vi "Prepare for a Scan_Load Settings.vi"(8 "error in (no error)":errorcluster, 11 "Command IN":string) -> (0 "error out":errorcluster)   [LabVIEW 2012]
doc: "SciScan 1.2 160622"
uses:
  INI/settingsIO/Settings IO_Commands.ctl
  MacroGUI Module/SubVIs/FGV_Macro Settings to GFG_Command.ctl
  Custom Controls/scan mode main settings tab.ctl
  image & display/Draw ROI on Line Scan Display Command.ctl
  Custom Controls/MAIN Image panel tab Control type def.ctl
  Custom Controls/advanced settings inner tab CTL.ctl
  System.Windows.Forms
panel:
  in  "Updating Settings...":refnum<k24>(container)
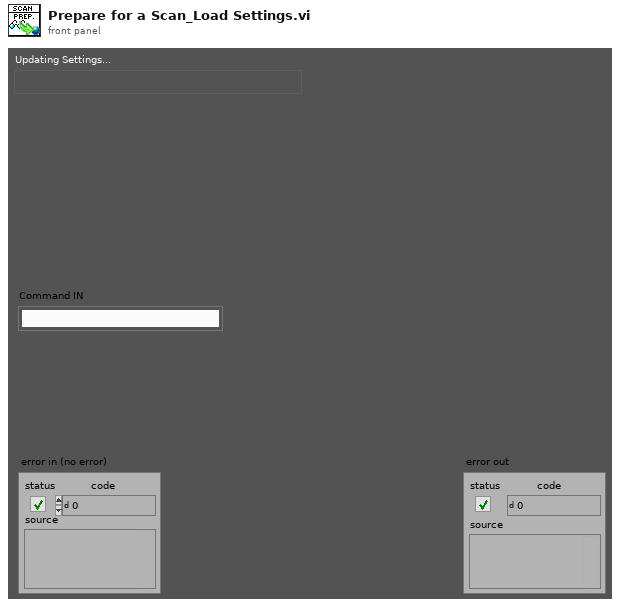
[diagram p1: front panel]
types:
  T1 = typedef "Setting File Types.ctl" = enum16{"2D.Frame.Scan.Settings", "2D.Line.Scan.Settings", "Z.Stack.Settings", "HW Settings", "Configuration Settings", "Unknown Settings", "Fast.Z.Settings"}
  T2 = typedef "scan mode main settings tab.ctl" = enum32{"2D frame", "2D line scan", "general settings", "Z Stack", "piezo"}
  T3 = typedef "FGV_Macro Settings to GFG_Command.ctl" = enum16{"Get Current Settings", "Backup Curent Settings", "Recover Backed up settings", "Overwrite Current Settings"}
  T4 = typedef "Settings IO_Commands.ctl" = enum16{"Write HW Settings", "Write Config Settings", "Read HW Settings", "Read Config Settings", "Write Line-Scan Settings", "Write Frame-Scan Settings", "Write Z-Stack Settings", "Read Line-Scan Settings", "Read Frame-Scan Settings", "Read Z-Stack Settings", "Read Fast-Z Settings", "Write Fast-Z Settings"}
  T5 = typedef "MAIN Image panel tab Control type def.ctl" = enum32{"Channel 1", "Channel 2", "Channel 3", "Channel 4", "all channels", "RGB overlay", "ROI", "arbitrary line scan"}
  T6 = typedef "Draw ROI on Line Scan Display Command.ctl" = enum16{"Draw ROI from GFG", "Clear ROI"}
  T7 = enum16{"Always Generate", "Generate if no valid image"}
  T8 = typedef "advanced settings inner tab CTL.ctl" = enum32{"arb. frames", "AO", "AI", "channels", "trigger", "Zstack data"}
  T9 = typedef "GFG Variable for IO.ctl" = cluster{"Variable Name":string, "Value (Variant)":variant, "data type":string}
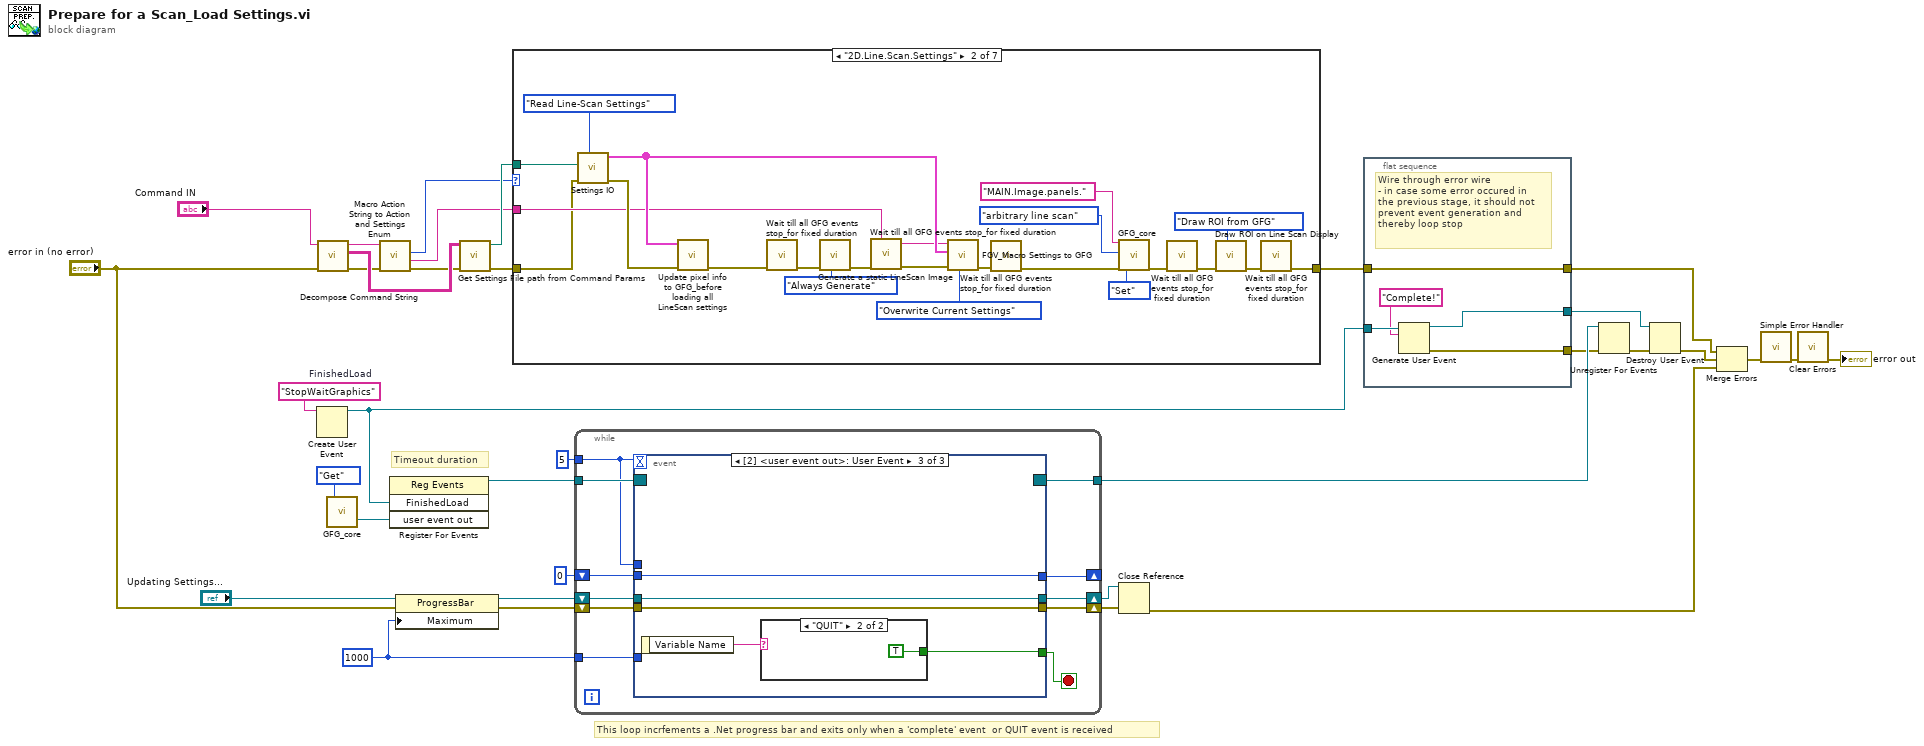
[diagram p0: block diagram]
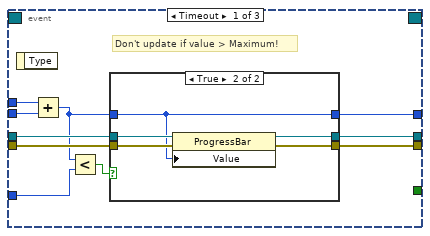
[diagram p2: hidden frame]
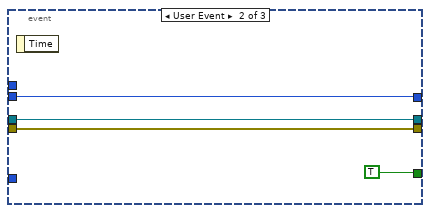
[diagram p4: hidden frame]
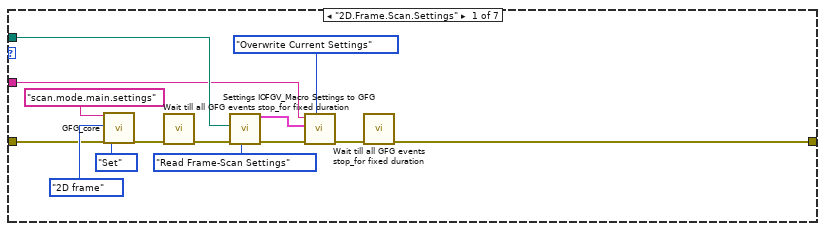
[diagram p6: hidden frame]
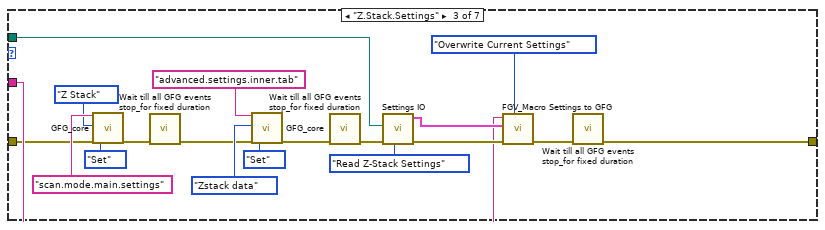
[diagram p7: hidden frame]
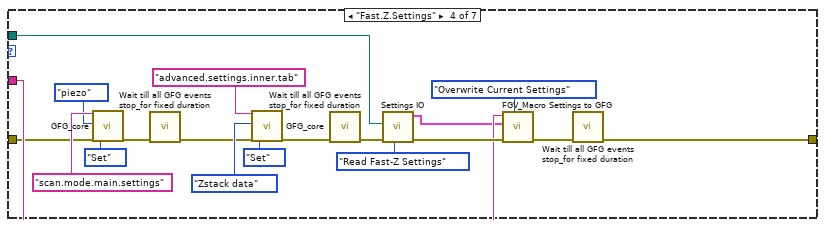
[diagram p8: hidden frame]
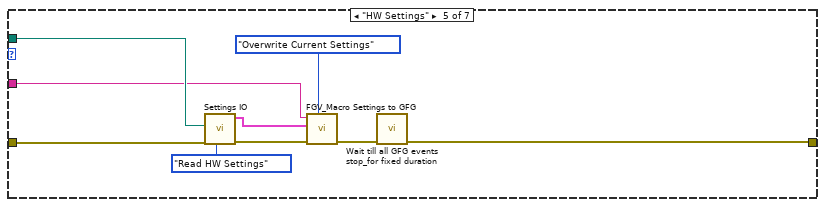
[diagram p9: hidden frame]
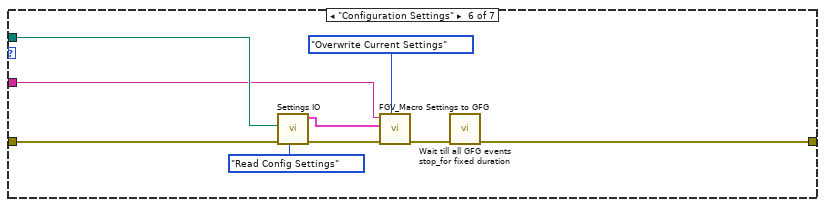
[diagram p10: hidden frame]
diagram:
  w12 = 1000 ("Maximum")
  w25 = "StopWaitGraphics"  # FinishedLoad
  # "This loop incrfements a .Net progress bar and exits only when a 'complete' event  or QUIT event is received"
  # "Timeout duration"
  n1 = Create User Event(user event datatype=w25) -> (user event=w22:refnum<user-event>)  [unwired: 1 in, 1 out]
  n2 = call "Decompose Command String.vi"("Error In"="error in (no error)", "Command IN"="Command IN") -> ("Error Out"=w33:errorcluster, "Parameter Table"=w34:string[][], "Action"=w32:string)  [unwired: 6 in, 1 out]
  n3 = call "GFG_core.vi"("Action"=enum16{"Init", "Set", "Get", "Clear"}."Get") -> ("user event out"=w1:refnum<user-event>)  [unwired: 12 in, 6 out]
  n4 = call "Macro Action String to Action and Settings Enum.vi"("error in (no error)"=w33, "Action String IN"=w32) -> ("error out"=w31:errorcluster, "Settings File Type OUT (String)"=w29:string, "Setting File Type OUT"=w28:T1)  [unwired: 6 in, 1 out]
  n5 = register-events(w22, w1) -> (reference out=w21:refnum<event-registration>)  [unwired: 2 in, 1 out]
  n6 = property class="ProgressBar"(reference="Updating Settings...", error in="error in (no error)", "Maximum"=w12) -> (reference out=w19:refnum<k24>, error out=w20:errorcluster)
  n7 = call "Get Settings File path from Command Params.vi"("error in (no error)"=w31, "Params Array IN"=w34) -> ("error out"=w26:errorcluster, "Settings Path OUT"=w30:path)  [unwired: 8 in]
  n8 = case shown="\"2D.Line.Scan.Settings\"" w28 {
    tunnel: [w43 w49 w82 w91 w109 w120 w127] -> w9
    tunnel: w30 -> [w42 w53 w84 w104 w111 w119 _]
    tunnel: w29 -> [w41 w52 w85 w105 w110 w118 _]
    tunnel: w26 -> [w37 w51 w75 w96 w112 w121 w127]
    frame "2D.Frame.Scan.Settings" {
      n9 = call "GFG_core.vi"("Variable Name in"="scan.mode.main.settings", "Variant in"=scan_mode_main_settings_tab."2D frame" ("scan mode main settings"), "error in (no error)"=w37, "Action"=enum16{"Init", "Set", "Get"}."Set") -> ("error out"=w36:errorcluster)  [unwired: 9 in, 6 out]
      n10 = call "Wait till all GFG events stop_for fixed duration.vi"("error in (no error)"=w36) -> ("error out"=w35:errorcluster)  [unwired: 10 in]
      n11 = call "Settings IO.vi"("SettingsFileIO_Commands"=Settings_IO_Commands."Read Frame-Scan Settings", "Error In"=w35, "File Path (for scan specific settings)"=w42) -> ("Error Out"=w46:errorcluster, "Settings Array OUT"=w45:T9[])  [unwired: 6 in, 1 out]
      n12 = call "FGV_Macro Settings to GFG.vi"("FGV_Macro Settings to GFG_Command"=FGV_Macro_Settings_to_GFG_Command."Overwrite Current Settings", "error in (no error)"=w46, "New Settings IN"=w45, "Settings type string IN"=w41) -> ("error out"=w44:errorcluster)  [unwired: 5 in, 2 out]
      n13 = call "Wait till all GFG events stop_for fixed duration.vi"("error in (no error)"=w44) -> ("error out"=w43:errorcluster)  [unwired: 10 in]
    }
    frame "2D.Line.Scan.Settings" {
      n14 = call "Settings IO.vi"("SettingsFileIO_Commands"=Settings_IO_Commands."Read Line-Scan Settings", "Error In"=w51, "File Path (for scan specific settings)"=w53) -> ("Error Out"=w68:errorcluster, "Settings Array OUT"=w67:T9[])  [unwired: 6 in, 1 out]
      n15 = call "Update pixel info to GFG_before loading all LineScan settings.vi"("error in (no error)"=w68, "All LineScan Settings IN"=w67) -> ("error out"=w66:errorcluster)  [unwired: 9 in]
      n16 = call "Wait till all GFG events stop_for fixed duration.vi"("error in (no error)"=w66) -> ("error out"=w64:errorcluster)  [unwired: 10 in]
      n17 = call "Generate a static LineScan Image.vi"("Generate Static Image Options"=T7."Always Generate", "error in (no error)"=w64) -> ("error out"=w59:errorcluster)  [unwired: 9 in]
      n18 = call "Wait till all GFG events stop_for fixed duration.vi"("error in (no error)"=w59) -> ("error out"=w58:errorcluster)  [unwired: 10 in]
      n19 = call "FGV_Macro Settings to GFG.vi"("FGV_Macro Settings to GFG_Command"=FGV_Macro_Settings_to_GFG_Command."Overwrite Current Settings", "error in (no error)"=w58, "New Settings IN"=w67, "Settings type string IN"=w52) -> ("error out"=w57:errorcluster)  [unwired: 5 in, 2 out]
      n20 = call "Wait till all GFG events stop_for fixed duration.vi"("error in (no error)"=w57) -> ("error out"=w54:errorcluster)  [unwired: 10 in]
      n21 = call "GFG_core.vi"("Variable Name in"="MAIN.Image.panels.", "Variant in"=MAIN_Image_panel_tab_Control_type_def."arbitrary line scan" ("MAIN Image panels"), "error in (no error)"=w54, "Action"=enum16{"Init", "Set", "Get"}."Set") -> ("error out"=w56:errorcluster)  [unwired: 9 in, 6 out]
      n22 = call "Wait till all GFG events stop_for fixed duration.vi"("error in (no error)"=w56) -> ("error out"=w55:errorcluster)  [unwired: 10 in]
      n23 = call "Draw ROI on Line Scan Display.vi"("Draw ROI on Line Scan Display_Command"=Draw_ROI_on_Line_Scan_Display_Command."Draw ROI from GFG", "error in (no error)"=w55) -> ("error out"=w50:errorcluster)  [unwired: 9 in]
      n24 = call "Wait till all GFG events stop_for fixed duration.vi"("error in (no error)"=w50) -> ("error out"=w49:errorcluster)  [unwired: 10 in]
    }
    frame "Z.Stack.Settings" {
      n25 = call "GFG_core.vi"("Variable Name in"="scan.mode.main.settings", "Variant in"=scan_mode_main_settings_tab."Z Stack" ("scan mode main settings"), "error in (no error)"=w75, "Action"=enum16{"Init", "Set", "Get"}."Set") -> ("error out"=w72:errorcluster)  [unwired: 9 in, 6 out]
      n26 = call "Wait till all GFG events stop_for fixed duration.vi"("error in (no error)"=w72) -> ("error out"=w73:errorcluster)  [unwired: 10 in]
      n27 = call "GFG_core.vi"("Variable Name in"="advanced.settings.inner.tab", "Variant in"=advanced_settings_inner_tab_CTL."Zstack data" ("advanced settings inner tab"), "error in (no error)"=w73, "Action"=enum16{"Init", "Set", "Get"}."Set") -> ("error out"=w74:errorcluster)  [unwired: 9 in, 6 out]
      n28 = call "Wait till all GFG events stop_for fixed duration.vi"("error in (no error)"=w74) -> ("error out"=w71:errorcluster)  [unwired: 10 in]
      n29 = call "Settings IO.vi"("SettingsFileIO_Commands"=Settings_IO_Commands."Read Z-Stack Settings", "Error In"=w71, "File Path (for scan specific settings)"=w84) -> ("Error Out"=w87:errorcluster, "Settings Array OUT"=w86:T9[])  [unwired: 6 in, 1 out]
      n30 = call "FGV_Macro Settings to GFG.vi"("FGV_Macro Settings to GFG_Command"=FGV_Macro_Settings_to_GFG_Command."Overwrite Current Settings", "error in (no error)"=w87, "New Settings IN"=w86, "Settings type string IN"=w85) -> ("error out"=w83:errorcluster)  [unwired: 5 in, 2 out]
      n31 = call "Wait till all GFG events stop_for fixed duration.vi"("error in (no error)"=w83) -> ("error out"=w82:errorcluster)  [unwired: 10 in]
    }
    frame "Fast.Z.Settings" {
      n32 = call "GFG_core.vi"("Variable Name in"="scan.mode.main.settings", "Variant in"=scan_mode_main_settings_tab."piezo" ("scan mode main settings"), "error in (no error)"=w96, "Action"=enum16{"Init", "Set", "Get"}."Set") -> ("error out"=w93:errorcluster)  [unwired: 9 in, 6 out]
      n33 = call "Wait till all GFG events stop_for fixed duration.vi"("error in (no error)"=w93) -> ("error out"=w94:errorcluster)  [unwired: 10 in]
      n34 = call "GFG_core.vi"("Variable Name in"="advanced.settings.inner.tab", "Variant in"=advanced_settings_inner_tab_CTL."Zstack data" ("advanced settings inner tab"), "error in (no error)"=w94, "Action"=enum16{"Init", "Set", "Get"}."Set") -> ("error out"=w95:errorcluster)  [unwired: 9 in, 6 out]
      n35 = call "Wait till all GFG events stop_for fixed duration.vi"("error in (no error)"=w95) -> ("error out"=w92:errorcluster)  [unwired: 10 in]
      n36 = call "Settings IO.vi"("SettingsFileIO_Commands"=Settings_IO_Commands."Read Fast-Z Settings", "Error In"=w92, "File Path (for scan specific settings)"=w104) -> ("Error Out"=w106:errorcluster, "Settings Array OUT"=w90:T9[])  [unwired: 6 in, 1 out]
      n37 = call "FGV_Macro Settings to GFG.vi"("FGV_Macro Settings to GFG_Command"=FGV_Macro_Settings_to_GFG_Command."Overwrite Current Settings", "error in (no error)"=w106, "New Settings IN"=w90, "Settings type string IN"=w105) -> ("error out"=w103:errorcluster)  [unwired: 5 in, 2 out]
      n38 = call "Wait till all GFG events stop_for fixed duration.vi"("error in (no error)"=w103) -> ("error out"=w91:errorcluster)  [unwired: 10 in]
    }
    frame "HW Settings" {
      n39 = call "Settings IO.vi"("SettingsFileIO_Commands"=Settings_IO_Commands."Read HW Settings", "Error In"=w112, "File Path (for scan specific settings)"=w111) -> ("Error Out"=w115:errorcluster, "Settings Array OUT"=w114:T9[])  [unwired: 6 in, 1 out]
      n40 = call "FGV_Macro Settings to GFG.vi"("FGV_Macro Settings to GFG_Command"=FGV_Macro_Settings_to_GFG_Command."Overwrite Current Settings", "error in (no error)"=w115, "New Settings IN"=w114, "Settings type string IN"=w110) -> ("error out"=w113:errorcluster)  [unwired: 5 in, 2 out]
      n41 = call "Wait till all GFG events stop_for fixed duration.vi"("error in (no error)"=w113) -> ("error out"=w109:errorcluster)  [unwired: 10 in]
    }
    frame "Configuration Settings" {
      n42 = call "Settings IO.vi"("SettingsFileIO_Commands"=Settings_IO_Commands."Read Config Settings", "Error In"=w121, "File Path (for scan specific settings)"=w119) -> ("Error Out"=w124:errorcluster, "Settings Array OUT"=w123:T9[])  [unwired: 6 in, 1 out]
      n43 = call "FGV_Macro Settings to GFG.vi"("FGV_Macro Settings to GFG_Command"=FGV_Macro_Settings_to_GFG_Command."Overwrite Current Settings", "error in (no error)"=w124, "New Settings IN"=w123, "Settings type string IN"=w118) -> ("error out"=w122:errorcluster)  [unwired: 5 in, 2 out]
      n44 = call "Wait till all GFG events stop_for fixed duration.vi"("error in (no error)"=w122) -> ("error out"=w120:errorcluster)  [unwired: 10 in]
    }
    frame "Unknown Settings", Default {
    }
  }
  n45 = while {
    shift-right: [w137] -> _
    shift-left: 0 -> [w138]
    tunnel: 5 -> [w129]
    tunnel: w21 -> [w136]
    shift-right: [w132] -> w17
    shift-left: w20 -> [w133]
    shift-right: [w131] -> w16
    shift-left: w19 -> [w135]
    tunnel: w12 -> [w130]
    tunnel: [w128] -> w6
    stop <- w134 stop-if-true
    n46 = event shown="[2] <user event out>: User Event" {
      selector: w136 -> [_ _ _]
      dyn-events: [_ _ _] -> w128
      timeout: w129 -> [_ _ _]
      tunnel: w138 -> [w141 w159 w165]
      tunnel: [w142 w159 w165] -> w137
      tunnel: w135 -> [w148 w157 w163]
      tunnel: [_ TRUE w161] -> w134
      tunnel: w133 -> [w147 w158 w164]
      tunnel: [w146 w158 w164] -> w132
      tunnel: [w145 w157 w163] -> w131
      tunnel: w130 -> [w143 _ _]
      tunnel: w129 -> [w139 _ _]
      event Timeout {
        # "Don't update if value > Maximum!"
        n47 = event-data() -> ()  [unwired: 1 in, 1 out]
        n48 = Add(x=w139, y=w141) -> (x+y=w140:i32)
        n49 = Less?(x=w140, y=w143) -> (x < y?=w144:bool)
        n50 = case shown="True" w144 {
          tunnel: w148 -> [w150 w156]
          tunnel: w147 -> [w151 w155]
          tunnel: w140 -> [w149 w152]
          tunnel: [w151 w154] -> w146
          tunnel: [w150 w153] -> w145
          tunnel: [w149 w152] -> w142
          frame False {
          }
          frame True {
            n51 = property class="ProgressBar"(reference=w156, error in=w155, "Value"=w152) -> (reference out=w153:refnum<k24>, error out=w154:errorcluster)
          }
        }
      }
      event User Event {
        n52 = event-data() -> ()  [unwired: 1 in, 1 out]
      }
      event User Event {
        n53 = event-data() -> ("Variable Name"=w162:string)  [unwired: 1 in]
        n54 = case shown="\"QUIT\"" w162 {
          tunnel: [_ TRUE] -> w161
          frame "False", Default {
          }
          frame "QUIT" {
          }
        }
      }
    }
  }
  n55 = Close Reference(reference=w16, error in (no error)=w17) -> (error out=w15:errorcluster)
  n56 = flat-sequence {
    tunnel: w22 -> [w171]
    tunnel: w9 -> [w167]
    tunnel: [w167] -> w3
    tunnel: [w169] -> w7
    tunnel: [w168] -> w5
    frame #0 {
      # "Wire through error wire\n- in case some error occured in \nthe previous stage, it should not \nprevent event generation and \nthereby loop stop"
      n57 = Generate User Event(user event=w171, event data cluster="Complete!" ("event data")) -> (user event out=w169:refnum<user-event>, error out=w168:errorcluster)  [unwired: 1 in]
    }
  }
  n58 = Unregister For Events(event registration refnum=w6, error in=w5) -> (error out=w8:errorcluster)
  n59 = Destroy User Event(user event=w7, error in=w8) -> (error out=w4:errorcluster)
  n60 = Merge Errors(w3, w4, w15) -> (w14:errorcluster)
  n61 = call <vilib>:"Simple Error Handler.vi"("error in (no error)"=w14) -> ("error out"=w11:errorcluster)  [unwired: 4 in, 4 out]
  n62 = call <vilib>:"Clear Errors.vi"("error in (no error)"=w11) -> ("error out"=→"error out":errorcluster)  [unwired: 6 in]
